vi "Init.vi"(8 "error in (no error)":errorcluster, 10 "index":i32, 11 "BC_Steady":refnum<class "NI_BC_Steady.lvclass">) -> (0 "error out":errorcluster, 3 "initialized BC_Steady":refnum<class "NI_BC_Steady.lvclass">)   [LabVIEW 2017, in "NI_PDE.lvlib" / "NI_BC_Steady.lvclass"]
uses:
  <vilib>/gmath/pde.llb/BCClass/BC_Steady/NI_BC_Steady.lvclass
  <vilib>/gmath/pde.llb/BCClass/Class Type.ctl
  <vilib>/gmath/pde.llb/Common/PDE_BC Type.ctl
  <vilib>/gmath/pde.llb/BCClass/NI_BC.lvclass
  <vilib>/gmath/NI_PDE.lvlib
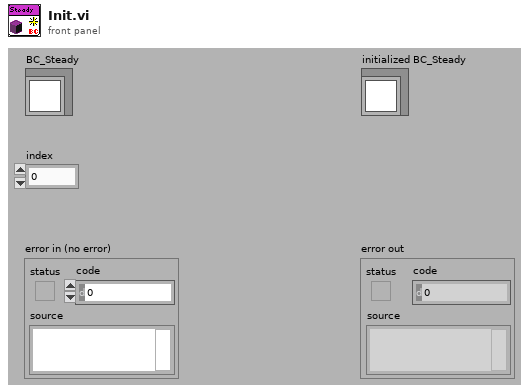
[diagram p1: front panel]
types:
  T1 = typedef "NI_PDE.lvlib/PDE_BC Type.ctl" = i32
  T2 = typedef "NI_PDE.lvlib/NI_BC.lvclass/Class Type.ctl" = i32
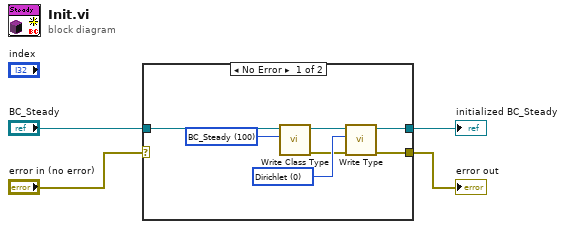
[diagram p0: block diagram]
diagram:
  n1 = case shown="No Error" "error in (no error)" {
    selector: "error in (no error)" -> [_ w13]
    tunnel: "BC_Steady" -> [w11 w12]
    tunnel: [w5 w13] -> w3
    tunnel: [w6 w12] -> w2
    frame No Error {
      w9 = T1 0 items=["Dirichlet", "Neumann"] ("BC type")
      w10 = T2 100 items=["BC"=0, "BC_Steady"=100, "BC_Steady_2D"=120, "BC_Steady_2D_Numeric"=121, "BC_Steady_2D_VIRef"=122, "BC_Evolut"=200, "BC_Evolut_1D"=210, "BC_Evolut_1D_Numeric"=211, "BC_Evolut_1D_VIRef"=212, "BC_Evolut_2D"=220, "BC_Evolut_2D_Numeric"=221, "BC_Evolut_2D_VIRef"=222] ("BC class type")
      n2 = call-dynamic "Write Class Type.vi"("BC class type"=w10, "BC.lvclass in"=w11) -> ("error out"=w7:errorcluster, "BC.lvclass out"=w8:refnum<class "NI_BC_Steady.lvclass">)  [unwired: 1 in, 7 out]
      n3 = call-dynamic "Write Type.vi"("error in (no error)"=w7, "BC type"=w9, "BC.lvclass in"=w8) -> ("error out"=w5:errorcluster, "BC.lvclass out"=w6:refnum<class "NI_BC_Steady.lvclass">)  [unwired: 7 out]
    }
    frame Error {
    }
  }
  "initialized BC_Steady" <- w2
  "error out" <- w3
